vi "Load Becker-Hickl Measurement FCS Information.vi"(8 "error in (no error)":errorcluster, 10 "Measurement FCS Info in":T1 {"FCS Type" format="%016.0f"; "FCS Decay Calc" format="%016b"}, 11 "string in":string) -> (0 "error out":errorcluster, 2 "Measurement FCS Info out":T1 {"FCS Type" format="%016.0f"; "FCS Decay Calc" format="%016b"}, 3 "string out":string)   [LabVIEW 2021, in "Becker-Hickl Files.lvlib"]
uses:
  Becker-Hickl Files.lvlib
  Becker-Hickl FCS Measurement Info.ctl
  Becker-Hickl Read Single U16.vi
  Becker-Hickl Read Single U32.vi
  Becker-Hickl Read Single SGL.vi
  Becker-Hickl Read Single I32.vi
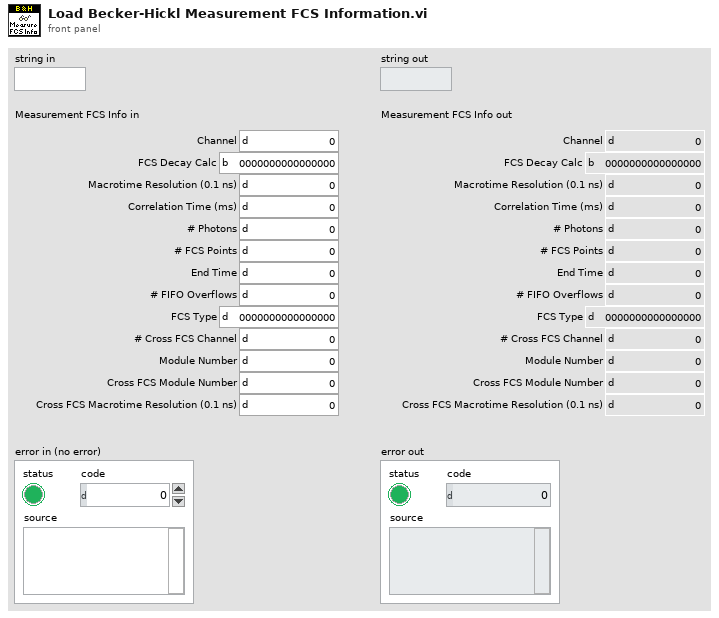
[diagram p1: front panel]
types:
  T1 = typedef "Becker-Hickl Files.lvlib/Becker-Hickl FCS Measurement Info.ctl" = cluster{"Channel":u16, "FCS Decay Calc":u16, "Macrotime Resolution (0.1 ns)":u32, "Correlation Time (ms)":sgl, "# Photons":u32, "# FCS Points":i32, "End Time":sgl, "# FIFO Overflows":u16, "FCS Type":u16, "# Cross FCS Channel":u16, "Module Number":u16, "Cross FCS Module Number":u16, "Cross FCS Macrotime Resolution (0.1 ns)":u32}
  T2 = enum16{"chan", "fcs_decay_calc", "mt_resol", "cortime", "calc_photons", "fcs_points", "end_time", "overruns", "fcs_type", "cross_chan", "mod", "cross_mod", "cross_mt_resol"}
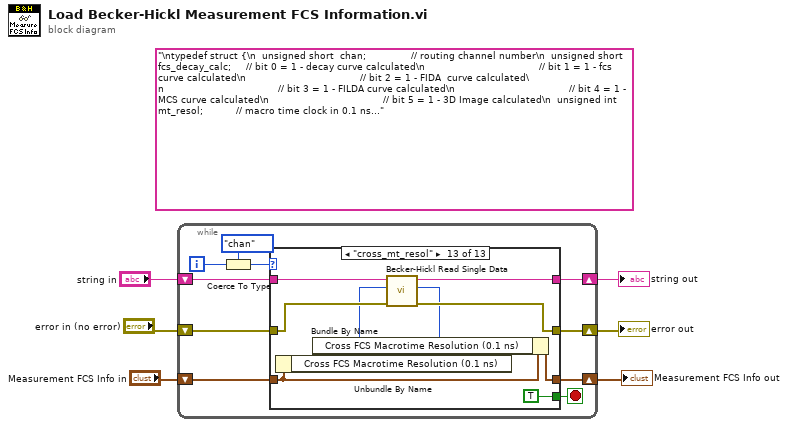
[diagram p0: block diagram]
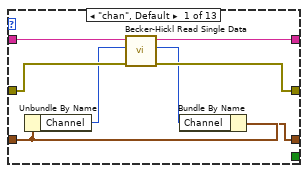
[diagram p2: hidden frame]
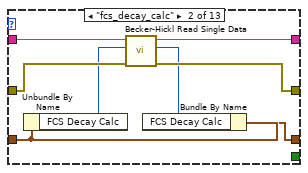
[diagram p3: hidden frame]
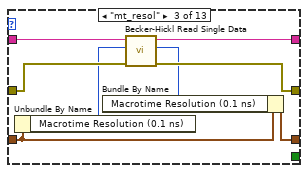
[diagram p4: hidden frame]
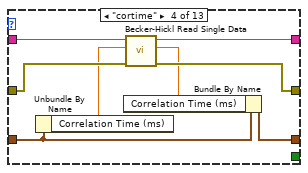
[diagram p5: hidden frame]
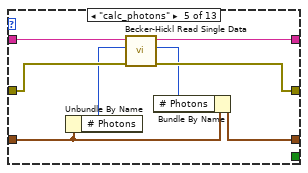
[diagram p6: hidden frame]
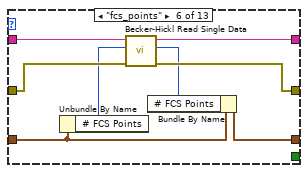
[diagram p7: hidden frame]
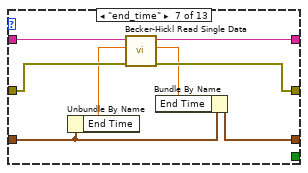
[diagram p8: hidden frame]
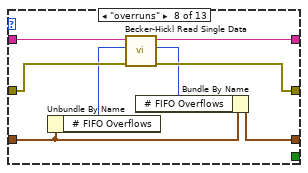
[diagram p9: hidden frame]
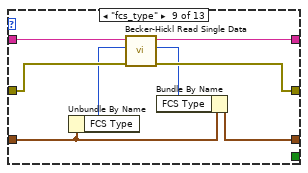
[diagram p10: hidden frame]
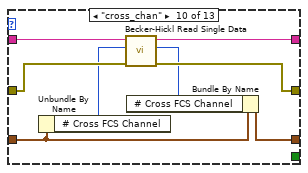
[diagram p11: hidden frame]
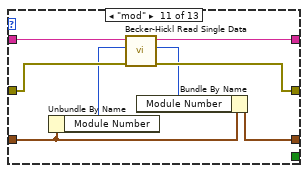
[diagram p12: hidden frame]
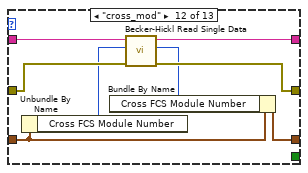
[diagram p13: hidden frame]
diagram:
  (unwired) "\ntypedef struct {\n  unsigned short  chan;               // routing channel number\n  unsigned short  fcs_decay_calc;     // bit 0 = 1 - decay curve calculated\n                                      // bit 1 = 1 - fcs   curve calculated\n                                      // bit 2 = 1 - FIDA  curve calculated\n                                      // bit 3 = 1 - FILDA curve calculated\n                                      // bit 4 = 1 - MCS curve calculated\n                                      // bit 5 = 1 - 3D Image calculated\n  unsigned int    mt_resol;           // macro time clock in 0.1 ns units\n  float           cortime;            // correlation time [ms] \n  unsigned int    calc_photons;       //  no of photons  \n  int             fcs_points;         // no of FCS values\n  float           end_time;           // macro time of the last photon \n  unsigned short  overruns;           // no of Fifo overruns \n                              //   when > 0  fcs curve & end_time are not valid\n  unsigned short  fcs_type;   // 0 - linear FCS with log binning ( 100 bins/log )\n                              // when bit 15 = 1 ( 0x8000 ) - Multi-Tau FCS \n                              //           where bits 14-0 = ktau parameter\n  unsigned short  cross_chan;         // cross FCS routing channel number\n                   //   when chan = cross_chan and mod == cross_mod - Auto FCS\n                   //        otherwise - Cross FCS\n  unsigned short  mod;                // module number\n  unsigned short  cross_mod;          // cross FCS module number\n  unsigned int    cross_mt_resol;     // macro time clock of cross FCS module in 0.1 ns units\n  }MeasFCSInfo;   // information collected when FIFO measurement is finished"
  n1 = while {
    shift-right: [w12] -> w5
    shift-left: "string in" -> [w15]
    shift-right: [w11] -> w3
    shift-left: "error in (no error)" -> [w14]
    shift-right: [w10] -> w1
    shift-left: "Measurement FCS Info in" -> [w13]
    i -> [w16]
    stop <- w7 stop-if-true
    n2 = Coerce To Type(0:w16, 1:T2."chan") -> (2:w9:T2)
    n3 = case shown="\"cross_mt_resol\"" w9 {
      tunnel: w15 -> [w24 w32 w40 w48 w56 w64 w72 w80 w88 w96 w104 w112 w121]
      tunnel: w14 -> [w21 w29 w37 w45 w53 w61 w69 w77 w85 w93 w101 w109 w118]
      tunnel: w13 -> [w20 w28 w36 w44 w52 w60 w68 w76 w84 w92 w100 w108 w117]
      tunnel: [w23 w31 w39 w47 w55 w63 w71 w79 w87 w95 w103 w111 w120] -> w12
      tunnel: [w22 w30 w38 w46 w54 w62 w70 w78 w86 w94 w102 w110 w119] -> w11
      tunnel: [w18 w26 w34 w42 w50 w58 w66 w74 w82 w90 w98 w106 w115] -> w10
      tunnel: [_ _ _ _ _ _ _ _ _ _ _ _ TRUE] -> w7
      frame "chan", Default {
        n4 = Unbundle By Name(w20) -> ("Channel"=w19:u16)
        n5 = call-poly "Becker-Hickl Read Single Data.vi"("Error In"=w21, "Default"=w19, "Bytes in"=w24) -> ("Error Out"=w22:errorcluster, "U16"=w17:u16, "Bytes out"=w23:string)  [unwired: 6 in]
        n6 = Bundle By Name(cluster=w20, "Channel"=w17) -> (w18:T1)
      }
      frame "fcs_decay_calc" {
        n7 = Unbundle By Name(w28) -> ("FCS Decay Calc"=w27:u16)
        n8 = call-poly "Becker-Hickl Read Single Data.vi"("Error In"=w29, "Default"=w27, "Bytes in"=w32) -> ("Error Out"=w30:errorcluster, "U16"=w25:u16, "Bytes out"=w31:string)  [unwired: 6 in]
        n9 = Bundle By Name(cluster=w28, "FCS Decay Calc"=w25) -> (w26:T1)
      }
      frame "mt_resol" {
        n10 = Unbundle By Name(w36) -> ("Macrotime Resolution (0.1 ns)"=w35:u32)
        n11 = call-poly "Becker-Hickl Read Single Data.vi"("Error In"=w37, "Default"=w35, "Bytes in"=w40) -> ("Error Out"=w38:errorcluster, "U32"=w33:u32, "Bytes out"=w39:string)  [unwired: 6 in]
        n12 = Bundle By Name(cluster=w36, "Macrotime Resolution (0.1 ns)"=w33) -> (w34:T1)
      }
      frame "cortime" {
        n13 = Unbundle By Name(w44) -> ("Correlation Time (ms)"=w43:sgl)
        n14 = call-poly "Becker-Hickl Read Single Data.vi"("Error In"=w45, "Default"=w43, "Bytes in"=w48) -> ("Error Out"=w46:errorcluster, "SGL"=w41:sgl, "Bytes out"=w47:string)  [unwired: 6 in]
        n15 = Bundle By Name(cluster=w44, "Correlation Time (ms)"=w41) -> (w42:T1)
      }
      frame "calc_photons" {
        n16 = Unbundle By Name(w52) -> ("# Photons"=w51:u32)
        n17 = call-poly "Becker-Hickl Read Single Data.vi"("Error In"=w53, "Default"=w51, "Bytes in"=w56) -> ("Error Out"=w54:errorcluster, "U32"=w49:u32, "Bytes out"=w55:string)  [unwired: 6 in]
        n18 = Bundle By Name(cluster=w52, "# Photons"=w49) -> (w50:T1)
      }
      frame "fcs_points" {
        n19 = Unbundle By Name(w60) -> ("# FCS Points"=w59:i32)
        n20 = call-poly "Becker-Hickl Read Single Data.vi"("Error In"=w61, "Default"=w59, "Bytes in"=w64) -> ("Error Out"=w62:errorcluster, "I32"=w57:i32, "Bytes out"=w63:string)  [unwired: 6 in]
        n21 = Bundle By Name(cluster=w60, "# FCS Points"=w57) -> (w58:T1)
      }
      frame "end_time" {
        n22 = Unbundle By Name(w68) -> ("End Time"=w67:sgl)
        n23 = call-poly "Becker-Hickl Read Single Data.vi"("Error In"=w69, "Default"=w67, "Bytes in"=w72) -> ("Error Out"=w70:errorcluster, "SGL"=w65:sgl, "Bytes out"=w71:string)  [unwired: 6 in]
        n24 = Bundle By Name(cluster=w68, "End Time"=w65) -> (w66:T1)
      }
      frame "overruns" {
        n25 = Unbundle By Name(w76) -> ("# FIFO Overflows"=w75:u16)
        n26 = call-poly "Becker-Hickl Read Single Data.vi"("Error In"=w77, "Default"=w75, "Bytes in"=w80) -> ("Error Out"=w78:errorcluster, "U16"=w73:u16, "Bytes out"=w79:string)  [unwired: 6 in]
        n27 = Bundle By Name(cluster=w76, "# FIFO Overflows"=w73) -> (w74:T1)
      }
      frame "fcs_type" {
        n28 = Unbundle By Name(w84) -> ("FCS Type"=w83:u16)
        n29 = call-poly "Becker-Hickl Read Single Data.vi"("Error In"=w85, "Default"=w83, "Bytes in"=w88) -> ("Error Out"=w86:errorcluster, "U16"=w81:u16, "Bytes out"=w87:string)  [unwired: 6 in]
        n30 = Bundle By Name(cluster=w84, "FCS Type"=w81) -> (w82:T1)
      }
      frame "cross_chan" {
        n31 = Unbundle By Name(w92) -> ("# Cross FCS Channel"=w91:u16)
        n32 = call-poly "Becker-Hickl Read Single Data.vi"("Error In"=w93, "Default"=w91, "Bytes in"=w96) -> ("Error Out"=w94:errorcluster, "U16"=w89:u16, "Bytes out"=w95:string)  [unwired: 6 in]
        n33 = Bundle By Name(cluster=w92, "# Cross FCS Channel"=w89) -> (w90:T1)
      }
      frame "mod" {
        n34 = Unbundle By Name(w100) -> ("Module Number"=w99:u16)
        n35 = call-poly "Becker-Hickl Read Single Data.vi"("Error In"=w101, "Default"=w99, "Bytes in"=w104) -> ("Error Out"=w102:errorcluster, "U16"=w97:u16, "Bytes out"=w103:string)  [unwired: 6 in]
        n36 = Bundle By Name(cluster=w100, "Module Number"=w97) -> (w98:T1)
      }
      frame "cross_mod" {
        n37 = Unbundle By Name(w108) -> ("Cross FCS Module Number"=w107:u16)
        n38 = call-poly "Becker-Hickl Read Single Data.vi"("Error In"=w109, "Default"=w107, "Bytes in"=w112) -> ("Error Out"=w110:errorcluster, "U16"=w105:u16, "Bytes out"=w111:string)  [unwired: 6 in]
        n39 = Bundle By Name(cluster=w108, "Cross FCS Module Number"=w105) -> (w106:T1)
      }
      frame "cross_mt_resol" {
        n40 = Unbundle By Name(w117) -> ("Cross FCS Macrotime Resolution (0.1 ns)"=w116:u32)
        n41 = call-poly "Becker-Hickl Read Single Data.vi"("Error In"=w118, "Default"=w116, "Bytes in"=w121) -> ("Error Out"=w119:errorcluster, "U32"=w114:u32, "Bytes out"=w120:string)  [unwired: 6 in]
        n42 = Bundle By Name(cluster=w117, "Cross FCS Macrotime Resolution (0.1 ns)"=w114) -> (w115:T1)
      }
    }
  }
  "Measurement FCS Info out" <- w1
  "error out" <- w3
  "string out" <- w5
